vi "GetNumThreads.vi"(8 "error in":errorcluster) -> (0 "error out":errorcluster, 3 "nThreads":i32)   [LabVIEW 2020, in "OpenLvVision_OpenCv.lvlib"]
doc: "Returns the number of threads used by OpenCV for parallel regions.\nAlways returns 1 if OpenCV is built without threading support."
uses:
  OpenLvVision_OpenCv.lvlib
  Dlls/OlvOpenCvWrapper.dll
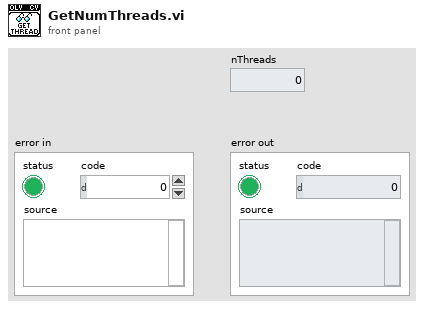
[diagram p1: front panel]
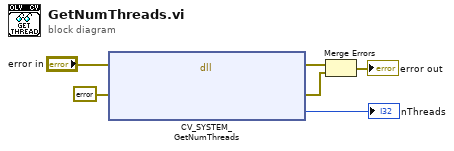
[diagram p0: block diagram]
diagram:
  n1 = dll-call lib="C:/Users/lukas/Downloads/OpenLvVision_OpenCv/SourceCode/LabView/OpenLvVision_OpenCv/Dlls/OlvOpenCvWrapper.dll" fn="CV_SYSTEM_GetNumThreads"(error in="error in", "Error"=errorcluster {"status"=FALSE, "code"=0, "source"=""} ("error in")) -> (error out=w4:errorcluster, "Error"=w2:errorcluster, "nThreads"=→"nThreads":i32)  [unwired: 4 in, 1 out]
  n2 = Merge Errors(w4, w2) -> (→"error out":errorcluster)
